vi "Periodic Tasks.vi"(8 "error in":errorcluster) -> ()   [LabVIEW 2015]
doc: "This VI runs in parallel to other robot code. It can contain as many user-defined periodic loops as you need. These can carry out PID or other sorts of timed response."
uses:
  <vilib>/Rock Robotics/WPI/Utilities/WPI_GetSetVariantRefNum.vi
  <vilib>/Rock Robotics/Network Tables/NT Write Numeric Array.vi
  Shooter/Implementation/Shooter Published Globals.vi
  <vilib>/Rock Robotics/Network Tables/NT Write Boolean.vi
  Robot Global Data.vi
  <vilib>/Rock Robotics/Network Tables/NT Write Number.vi
  Support Code/navX Library v2/navX Library v2.lvlib
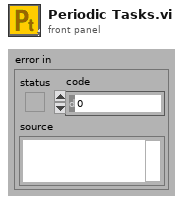
[diagram p1: front panel]
types:
  T1 = typedef "navX Library v2.lvlib/Z900_navX_DeviceTypeDef.ctl" = cluster{"Interface":cluster{"Protocol":T2, "Update Rate (4Hz-60Hz)":u8, "navX Open TypeDef":variant}, "Notify Packet":refnum<notifier>, "Loop VI Refnum":refnum<vi>, "Ready to Close Occurrence Refnum":refnum<k4>}
  T2 = typedef "navX Library v2.lvlib/Z900_navX_ProtocolTypeDef.ctl" = enum16{"SERIAL", "I2C", "SPI"}
  T3 = typedef "WPI_JoystickDevRef.ctl" = cluster{"Device":T4}
  T4 = typedef "WPI_JoystickDeviceEnum.ctl" = enum16{"USB 0", "USB 1", "USB 2", "USB 3", "USB 4", "USB 5"}
  T5 = cluster{"Yaw":dbl, "Roll":dbl, "Pitch":dbl, "Heading":dbl, "Fused Heading":dbl}
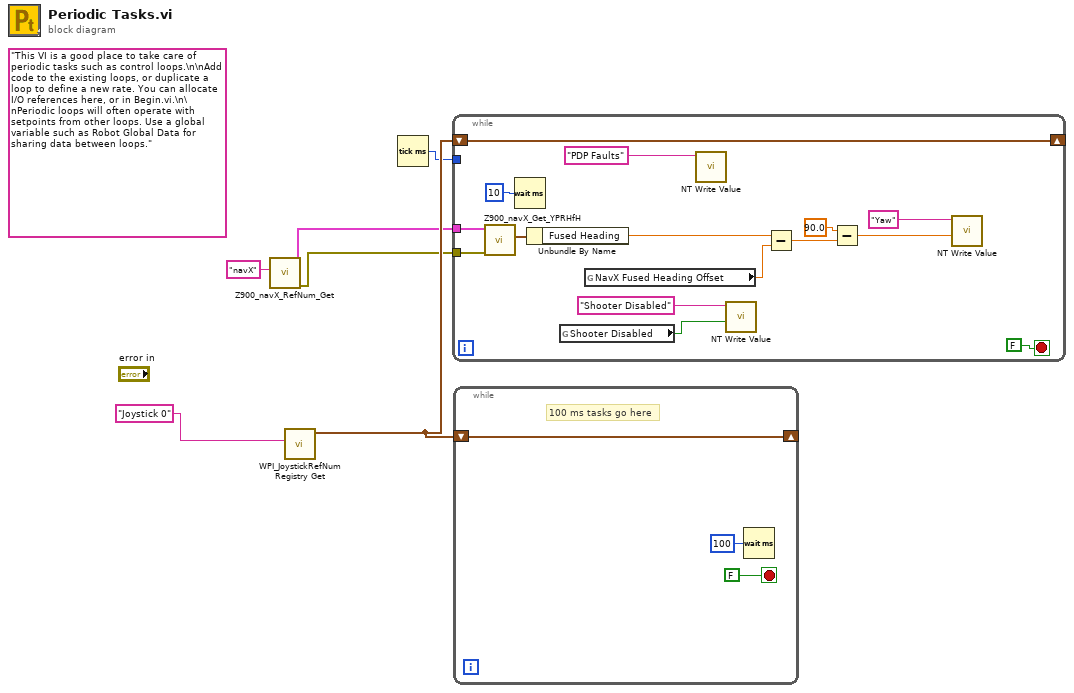
[diagram p0: block diagram]
diagram:
  (unwired) "This VI is a good place to take care of periodic tasks such as control loops.\n\nAdd code to the existing loops, or duplicate a loop to define a new rate. You can allocate I/O references here, or in Begin.vi.\n\nPeriodic loops will often operate with setpoints from other loops. Use a global variable such as Robot Global Data for sharing data between loops."
  n1 = call "Z900_navX_RefNum_Get.vi"("refnum name"="navX") -> ("error out"=w1:errorcluster, "navX Device"=w2:T1)  [unwired: 9 in]
  n2 = call <vilib>:"WPI_JoystickRefNum Registry Get.vi"("refnum name"="Joystick 0") -> ("JoystickDevRef"=w5:T3)  [unwired: 1 in, 9 out]
  n3 = Tick Count (ms)() -> (millisecond timer value=w4:u32)
  n4 = while {
    shift-right: [w20] -> _
    shift-left: w5 -> [w20]
    tunnel: w4 -> [_]
    tunnel: w2 -> [w9]
    tunnel: w1 -> [w8]
    stop <- FALSE stop-if-true
    n5 = call "Z900_navX_Get_YPRHfH.vi"("error in (no error)"=w8, "navX Device"=w9) -> ("YRPHfH"=w7:T5)  [unwired: 6 in, 3 out]
    n6 = Wait (ms)(milliseconds to wait=u32 10) -> ()  [unwired: 1 out]
    n7 = Unbundle By Name(w7) -> ("Fused Heading"=w12:dbl)
    n8 = global read "Shooter Published Globals.vi" "Shooter Disabled"() -> (w16:bool)
    n9 = global read "Robot Global Data.vi" "NavX Fused Heading Offset"() -> (w11:dbl)
    n10 = call-poly <vilib>:"NT Write Value.vi"("Name"="PDP Faults") -> ()  [unwired: 10 in, 1 out]
    n11 = call-poly <vilib>:"NT Write Value.vi"("Boolean"=w16, "Name"="Shooter Disabled") -> ()  [unwired: 9 in, 1 out]
    n12 = Subtract(x=w12, y=w11) -> (x-y=w10:dbl)
    n13 = Subtract(x=90.0, y=w10) -> (x-y=w14:dbl)
    n14 = call-poly <vilib>:"NT Write Value.vi"("Numeric"=w14, "Name"="Yaw") -> ()  [unwired: 9 in, 1 out]
  }
  n15 = while {
    shift-right: [w22] -> _
    shift-left: w5 -> [w22]
    stop <- FALSE stop-if-true
    # "100 ms tasks go here"
    n16 = Wait (ms)(milliseconds to wait=u32 100) -> ()  [unwired: 1 out]
  }
